vi "GetFPObjTypes.vi"(8 "error in (no error)":errorcluster, 11 "Object Reference":refnum<vi>) -> (0 "error out":errorcluster, 2 "Object Type":string, 3 "reference out":refnum<vi>)   [LabVIEW 2016]
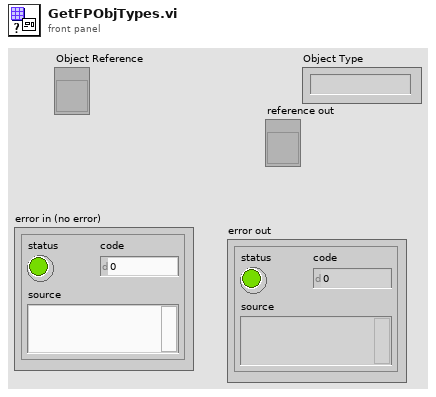
[diagram p1: front panel]
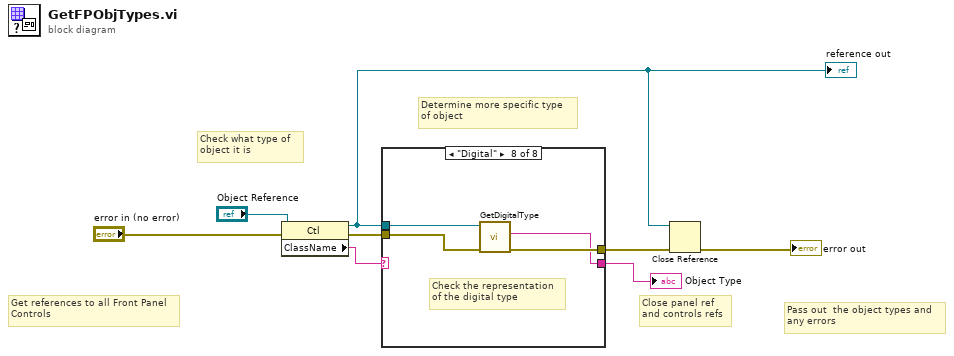
[diagram p0: block diagram]
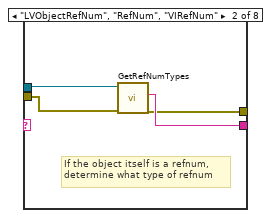
[diagram p3: hidden frame]
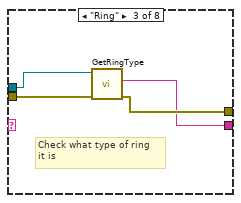
[diagram p4: hidden frame]
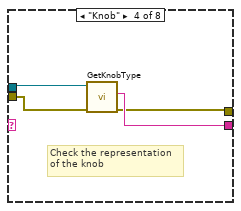
[diagram p5: hidden frame]
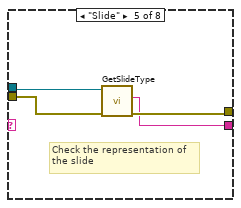
[diagram p6: hidden frame]
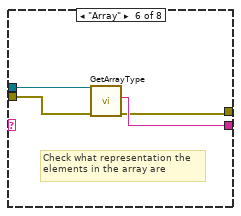
[diagram p7: hidden frame]
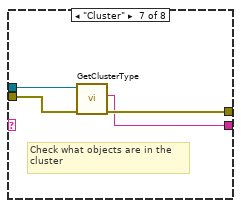
[diagram p8: hidden frame]
diagram:
  # "Determine more specific type\nof object"
  # "Check what type of\nobject it is"
  # "Close panel ref\nand controls refs"
  # "Get references to all Front Panel\nControls"
  # "Pass out  the object types and\nany errors"
  n1 = property class="Ctl"(reference="Object Reference", error in="error in (no error)") -> (reference out=w3:refnum<vi>, error out=w6:errorcluster, "ClassName"=w7:string)
  "reference out" <- w3
  n2 = case shown="\"Digital\"" w7 {
    selector: w7 -> [w9 _ _ _ _ _ _ _]
    tunnel: w3 -> [_ w13 w17 w19 w26 w30 w34 w37]
    tunnel: w6 -> [w10 w14 w18 w22 w25 w29 w33 w38]
    tunnel: [w9 w12 w15 w21 w23 w28 w31 w35] -> w5
    tunnel: [w10 w11 w16 w20 w24 w27 w32 w36] -> w8
    frame Default {
      # "If other object, just pass through\nclass name"
    }
    frame "LVObjectRefNum", "RefNum", "VIRefNum" {
      # "If the object itself is a refnum,\ndetermine what type of refnum"
      n3 = call "GetRefNumTypes.vi"("error in (no error)"=w14, "Control in"=w13) -> ("error out"=w11:errorcluster, "RefNumType"=w12:string)  [unwired: 7 in, 1 out]
    }
    frame "Ring" {
      # "Check what type of ring\nit is"
      n4 = call "GetRingType.vi"("error in (no error)"=w18, "Control Ref In"=w17) -> ("error out"=w16:errorcluster, "Ring Type"=w15:string)  [unwired: 7 in, 1 out]
    }
    frame "Knob" {
      # "Check the representation\nof the knob"
      n5 = call "GetKnobType.vi"("error in (no error)"=w22, "reference in"=w19) -> ("error out"=w20:errorcluster, "Knob Type"=w21:string)  [unwired: 7 in, 1 out]
    }
    frame "Slide" {
      # "Check the representation of\nthe slide"
      n6 = call "GetSlideType.vi"("error in (no error)"=w25, "Control in"=w26) -> ("error out"=w24:errorcluster, "Knob Type"=w23:string)  [unwired: 7 in, 1 out]
    }
    frame "Array" {
      # "Check what representation the\nelements in the array are"
      n7 = call "GetArrayType.vi"("error in (no error)"=w29, "Control in"=w30) -> ("error out"=w27:errorcluster, "Type"=w28:string)  [unwired: 7 in, 1 out]
    }
    frame "Cluster" {
      # "Check what objects are in the \ncluster"
      n8 = call "GetClusterType.vi"("error in"=w33, "Control in"=w34) -> ("error out"=w32:errorcluster, "Cluster Type"=w31:string)  [unwired: 7 in, 1 out]
    }
    frame "Digital" {
      # "Check the representation\nof the digital type"
      n9 = call "GetDigitalType.vi"("error in (no error)"=w38, "Control in"=w37) -> ("error out"=w36:errorcluster, "String"=w35:string)  [unwired: 7 in, 1 out]
    }
  }
  "Object Type" <- w5
  n10 = Close Reference(reference=w3, error in (no error)=w8) -> (error out=→"error out":errorcluster)
